vi "Comm_open 1d cdb waveform.vi"(6 "Access":T2, 7 "Communication Properties":T1={"WPL"={"Custom Queue Size"=1, "Use Custom Queue Size?"=FALSE}}, 8 "error in (no error)":errorcluster, 9 "dt":dbl=nan, 10 "Waveform Data Refs":i32[](array[numeric]), 11 "WPL Comm (1D CDB) in":refnum<class "WPL Comm (1D CDB).lvclass">) -> (0 "error out":errorcluster, 3 "WPL Comm (1D CDB) out":refnum<class "WPL Comm (1D CDB).lvclass">)   [LabVIEW 2020, in "Internal Comm Classes.lvlib" / "WPL Comm (1D CDB).lvclass"]
uses:
  WPL Comm (1D CDB).lvclass
  D:/p4/penguin/lvaddon/Veristand/master/src/LabVIEW/vilib/NI VeriStand/Custom Device Waveform API/Internal Comm Classes/WPL Comm/WPL Comm.lvclass
  Access mode.ctl
  Communication Properties.ctl
  WPL Comm (1D CDB).lvclass/WPL Comm (1D CDB).ctl
  Waveform 1d cdb read cluster.ctl
  Waveform properties.ctl
  Custom Device API/Waveform Data Reference.ctl
  WPL Command.ctl
  WPL Comm.lvclass/WPL Comm.ctl
  Send WPL Command.vi
  Set ErrorQ on Variant.vi
  Set dt on Variant.vi
  Error Check Empty Ref Array.vi
  Convert Q Error to Shutdown Error.vi
  <vilib>/Utility/error.llb/Error Cluster From Error Code.vi
  WPL Comm.lvclass
  NI_VS Custom Device Waveform API.lvlib
  Custom Device API/Custom Device API.lvlib
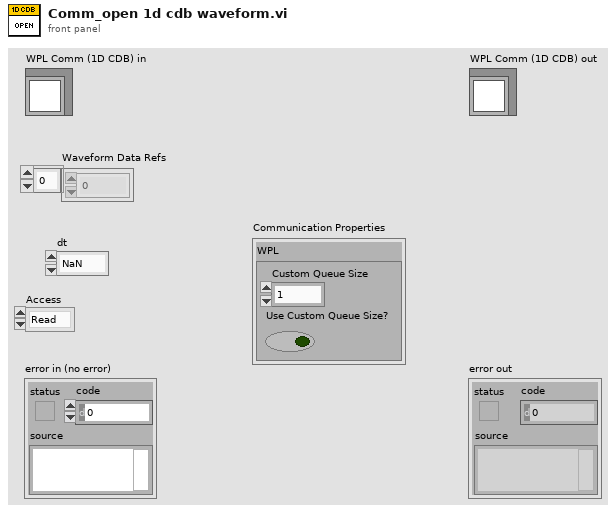
[diagram p1: front panel]
types:
  T1 = typedef "NI_VS Custom Device Waveform API.lvlib/Communication Properties.ctl" = cluster{"WPL":cluster{"Custom Queue Size":i32, "Use Custom Queue Size?":bool}}
  T2 = typedef "NI_VS Custom Device Waveform API.lvlib/Access mode.ctl" = enum16{"Read", "Write"}
  T3 = typedef "Internal Comm Classes.lvlib/WPL Comm (1D CDB).lvclass/Waveform 1d cdb read cluster.ctl" = cluster{"Waveform Properties":T4, "Data":cdb[]}
  T4 = typedef "NI_VS Custom Device Waveform API.lvlib/Waveform properties.ctl" = cluster{"Data reference":T5, "t0 at start":timestamp, "dt":dbl, "offset from start (samples)":u64}
  T5 = typedef "Custom Device API.lvlib/Waveform Data Reference.ctl" = i32
  T6 = typedef "Internal Comm Classes.lvlib/WPL Comm.lvclass/WPL Command.ctl" = enum16{"Register 1D DBL Reader", "Unregister 1D DBL Reader", "Register 1D DBL Writer", "Register 2D DBL Writer", "Unregister 1D DBL Writer", "Unregister 2D DBL Writer", "DBL WFM Start", "WFM 1D DBL Data", "WFM 2D DBL Data", "Shut down", "Handle Error", "Register 1D CDB Reader", "Unregister 1D CDB Reader", "Register 1D CDB Writer", "Unregister 1D CDB Writer", "Register 2D CDB Writer", "Unregister 2D CDB Writer", "WFM 1D CDB Data", "WFM 2D CDB Data", "CDB WFM Start", "Error Shutdown", "Register Streams", "Unregister Streams", "Delete All Streams", "Get WFM DTs", "DBL WFM Multi Start", "CDB WFM Multi Start"}
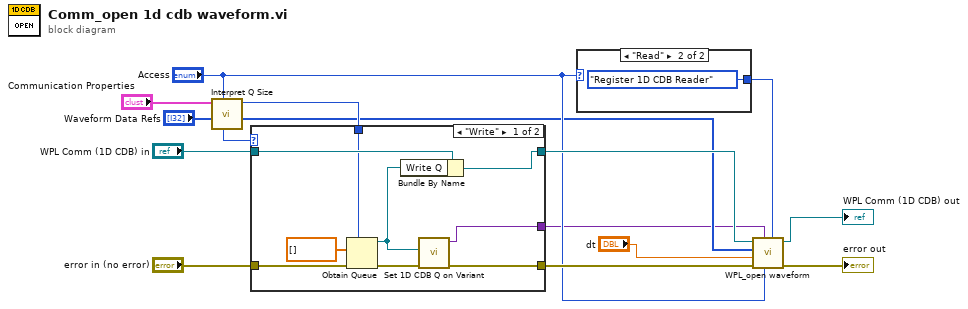
[diagram p0: block diagram]
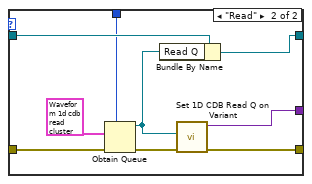
[diagram p2: hidden frame]
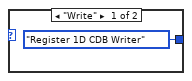
[diagram p3: hidden frame]
diagram:
  n1 = call "Interpret Q Size.vi"("Access"="Access", "Waveform Data References"="Waveform Data Refs", "Communication Properties"="Communication Properties") -> ("Waveform Data References dup"=w3:i32[], "Queue Size"=w7:i32, "Access dup"=w5:T2)  [unwired: 6 in]
  n2 = case shown="\"Write\"" w5 {
    tunnel: "error in (no error)" -> [w24 w33]
    tunnel: "WPL Comm (1D CDB) in" -> [w23 w32]
    tunnel: [w20 w30] -> w10
    tunnel: [w19 w29] -> w9
    tunnel: w7 -> [w18 w28]
    tunnel: [w16 w25] -> w1
    frame "Write" {
      n3 = Obtain Queue(max queue size (-1, unlimited)=w18, element data type=cdb[] [], error in (no error)=w24) -> (queue out=w17:refnum<queue>, error out=w21:errorcluster)  [unwired: 2 in, 1 out]
      n4 = Bundle By Name(cluster=w23, "Write Q"=w17) -> (w20:refnum<class "WPL Comm (1D CDB).lvclass">)
      n5 = call "Set 1D CDB Q on Variant.vi"("error in (no error)"=w21, "1D CDB Data Q"=w17) -> ("error out"=w19:errorcluster, "Variant out"=w16:variant)  [unwired: 7 in, 1 out]
    }
    frame "Read" {
      n6 = Obtain Queue(max queue size (-1, unlimited)=w28, element data type=T3 {"Waveform Properties"={"Data reference"=0, "t0 at start"=timestamp(0 s since 1904-01-01), "dt"=0.0, "offset from start (samples)"=0}, "Data"=[]} ("Read Cluster"), error in (no error)=w33) -> (queue out=w26:refnum<queue>, error out=w31:errorcluster)  [unwired: 2 in, 1 out]
      n7 = Bundle By Name(cluster=w32, "Read Q"=w26) -> (w30:refnum<class "WPL Comm (1D CDB).lvclass">)
      n8 = call "Set 1D CDB Read Q on Variant.vi"("error in (no error)"=w31, "1D CDB Read Q"=w26) -> ("error out"=w29:errorcluster, "Variant out"=w25:variant)  [unwired: 7 in, 1 out]
    }
  }
  n9 = case shown="\"Read\"" "Access" {
    tunnel: [WPL_Command."Register 1D CDB Writer" ("Command") WPL_Command."Register 1D CDB Reader" ("Command")] -> w2
    frame "Write" {
    }
    frame "Read" {
    }
  }
  n10 = call "WPL_open waveform.vi"("Command"=w2, "Access"="Access", "Variant in"=w1, "error in (no error)"=w9, "dt"="dt", "WFM Data Idx"=w3, "WPL Comm in"=w10) -> ("error out"=→"error out":errorcluster, "WPL Comm out"=→"WPL Comm (1D CDB) out":refnum<class "WPL Comm (1D CDB).lvclass">)  [unwired: 3 in]
